vi "smooth.vi"(0 "data":dbl format="%.2f", 1 "samples to average":u32, 2 "reset":bool) -> (7 "smoothed data":dbl format="%.2f", 8 "standard deviation":dbl format="%.2f")   [LabVIEW 2010]
uses:
  <vilib>/Analysis/NI_AALBase.lvlib
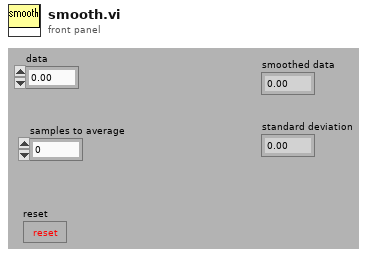
[diagram p1: front panel]
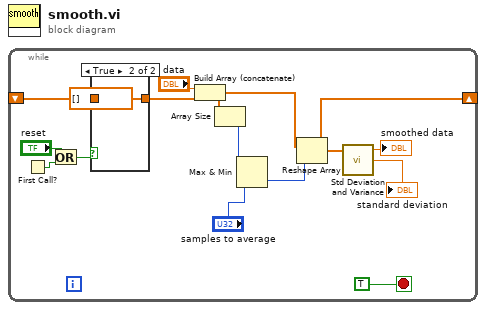
[diagram p0: block diagram]
diagram:
  n1 = while {
    shift-left: _ -> [w14]
    shift-right: [w10] -> _
    stop <- TRUE stop-if-true
    n2 = First Call?() -> (First Call?: T/F=w3:bool)
    n3 = Or(x="reset", y=w3) -> (x .or. y?=w1:bool)
    n4 = case shown="True" w1 {
      tunnel: w14 -> [w15 _]
      tunnel: [w15 dbl[] []] -> w12
      frame False {
      }
      frame True {
      }
    }
    n5 = Build Array (concatenate)("data", w12) -> (w11:dbl[])
    n6 = Array Size(array=w11) -> (size(s)=w6:i32)
    n7 = Max & Min(x=w6, y="samples to average") -> (min(x,y)=w4:u32)  [unwired: 1 out]
    n8 = Reshape Array(w11, w4) -> (w10:dbl[])
    n9 = call <vilib>:"Std Deviation and Variance.vi"("X"=w10) -> ("mean"=→"smoothed data":dbl, "standard deviation"=→"standard deviation":dbl)  [unwired: 1 in, 1 out]
  }
